vi "Producer Console Entry.vi"(0 "Prod-Data In":T2={"Queue_Producer"=refnum, "Queue_Consumer"=refnum, "To_GUI-Error_message"=refnum, "Rx-Data"=[], "Tx-Data"=[], "Console log"="", "Communication Settings"={"Tx Protocol"=enum."Not Active", "Rx Protocol"=enum."Serial", "Serial"={"Tx Port"="", "Rx Port"="", "Baud rate"=8, "Parity"=enum."Space", "Data bits"=0, "Stop bits"=0, "Flow control"=enum."None", "Tx Resource"="", "Rx Resource"=""}, "MIDI Device"={"Input uDevice ID"=0, "Output uDevice ID"=0, "hmidiout Handle"=0, "hmidiin Handle"=0}, "Bluetooth"={"Dummy"=""}, "USB"={"Dummy"=""}}, "MIDI-Messages"=[], "Queue_Session"=refnum, "To_GUI-Pre-Session"=refnum, "To_GUI-Producer"=refnum, "Tx Info"={"Datatype"=[], "Bytesize"=[], "Strings"=[], "ByteSum"=0}, "Payload"=variant, "Timout-Time[ms]"=0, "To_GUI-Session"=refnum, "CPU(ms)"=0}, 11 "Console Entry":string, 13 "Error In":errorcluster) -> (4 "Prod-Data Out":T2={"Queue_Producer"=refnum, "Queue_Consumer"=refnum, "To_GUI-Error_message"=refnum, "Rx-Data"=[], "Tx-Data"=[], "Console log"="", "Communication Settings"={"Tx Protocol"=enum."Not Active", "Rx Protocol"=enum."Serial", "Serial"={"Tx Port"="", "Rx Port"="", "Baud rate"=8, "Parity"=enum."Space", "Data bits"=0, "Stop bits"=0, "Flow control"=enum."None", "Tx Resource"="", "Rx Resource"=""}, "MIDI Device"={"Input uDevice ID"=0, "Output uDevice ID"=0, "hmidiout Handle"=0, "hmidiin Handle"=0}, "Bluetooth"={"Dummy"=""}, "USB"={"Dummy"=""}}, "MIDI-Messages"=[], "Queue_Session"=refnum, "To_GUI-Pre-Session"=refnum, "To_GUI-Producer"=refnum, "Tx Info"={"Datatype"=[], "Bytesize"=[], "Strings"=[], "ByteSum"=0}, "Payload"=variant, "Timout-Time[ms]"=0, "To_GUI-Session"=refnum, "CPU(ms)"=0})   [LabVIEW 2019]
doc: "Adds a new entry to a console log, if an error has occured it will also be logged."
uses:
  Controls/Producer-Data.ctl
  Common/Controls/Application_Message.ctl
  Common/Controls/Application_State.ctl
  Common/Controls/Communication_Settings.ctl
  Common/Controls/Communication_Protocols.ctl
  MIDI/Controls/MIDI-Message_Array.ctl
  MIDI/Controls/MIDI-Message_Cluster.ctl
  MIDI/Controls/Meta_Commands.ctl
  Controls/Prod - Tx_Info.ctl
panel:
  in  "Tab Control":T1(tab)
  out "Console log in":string
  out "Timestamp":string
  out "Console log out":string
  out "VI-filename":string
  out "VI Path":path
  out "Code Size":u32
  out "Revision Number":u32
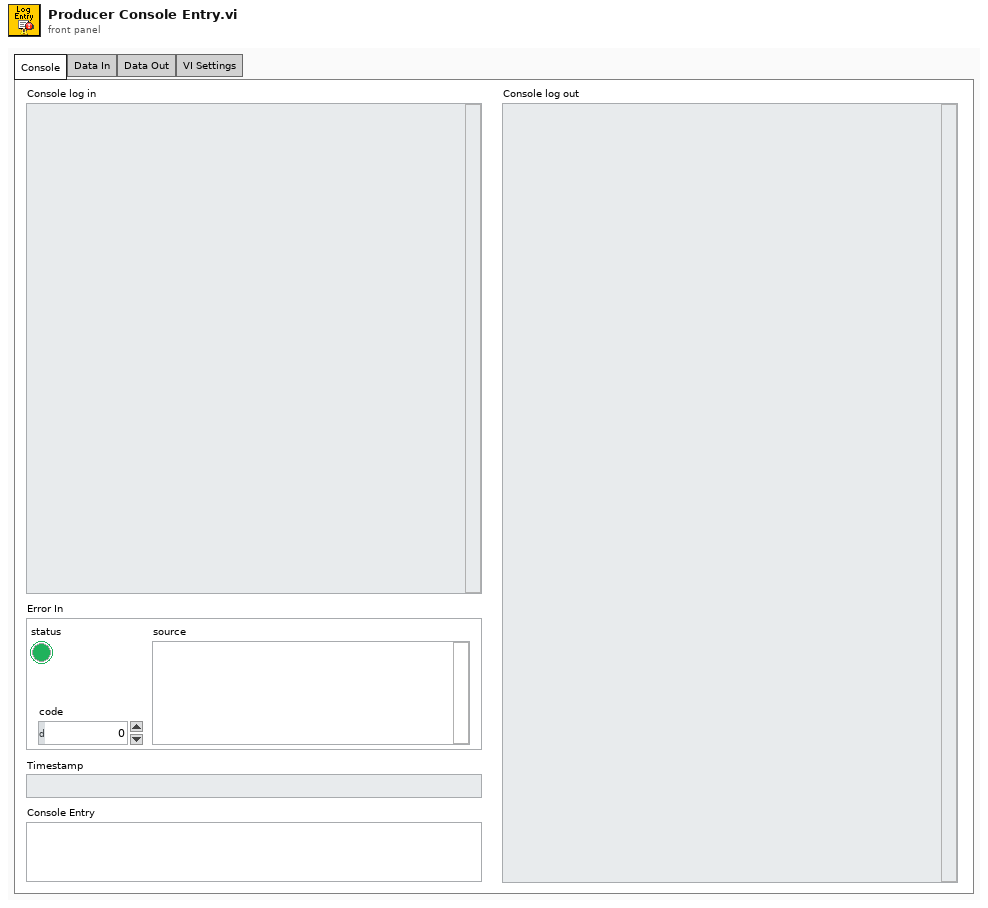
[diagram p1: front panel]
types:
  T1 = enum32{"Console", "Data In", "Data Out", "VI Settings"}
  T2 = typedef "Producer-Data.ctl" = cluster{"Queue_Producer":refnum<queue>, "Queue_Consumer":refnum<queue>, "To_GUI-Error_message":refnum<user-event>, "Rx-Data":i8[], "Tx-Data":i8[], "Console log":string, "Communication Settings":T3, "MIDI-Messages":T5, "Queue_Session":refnum<queue>, "To_GUI-Pre-Session":refnum<user-event>, "To_GUI-Producer":refnum<user-event>, "Tx Info":T8, "Payload":variant, "Timout-Time[ms]":i32, "To_GUI-Session":refnum<user-event>, "CPU(ms)":u32}
  T3 = typedef "Communication_Settings.ctl" = cluster{"Tx Protocol":T4, "Rx Protocol":T4, "Serial":cluster{"Tx Port":refnum<visa-resource-name>, "Rx Port":refnum<visa-resource-name>, "Baud rate":i32, "Parity":enum16{"None", "Odd", "Even", "Mark", "Space"}, "Data bits":i32, "Stop bits":i32, "Flow control":enum16{"None", "XON/XOFF", "RTS/CTS", "XON/XOFF & RTS/CTS", "DTR/DSR", "XON/XOFF & DTR/DSR"}, "Tx Resource":refnum<visa-resource-name>, "Rx Resource":refnum<visa-resource-name>}, "MIDI Device":cluster{"Input uDevice ID":u32, "Output uDevice ID":u32, "hmidiout Handle":i32, "hmidiin Handle":i32}, "Bluetooth":cluster{"Dummy":string}, "USB":cluster{"Dummy":string}}
  T4 = typedef "Communication_Protocols.ctl" = enum16{"Serial", "Bluetooth", "USB-MIDI", "MIDI (Audio Device)", "Not Active"}
  T5 = typedef "MIDI-Message_Array.ctl" = T6[]
  T6 = typedef "MIDI-Message_Cluster.ctl" = cluster{"Message Name":string, "Meta value":i32, "Datastring":string, "Datatype":T7}
  T7 = typedef "Meta_Commands.ctl" = enum16{"No Data", "Pause", "Loop", "Wait for Rx", "Delay", "Break", "MIDI"}
  T8 = typedef "Prod - Tx_Info.ctl" = cluster{"Datatype":T7[], "Bytesize":i32[], "Strings":string[], "ByteSum":i32}
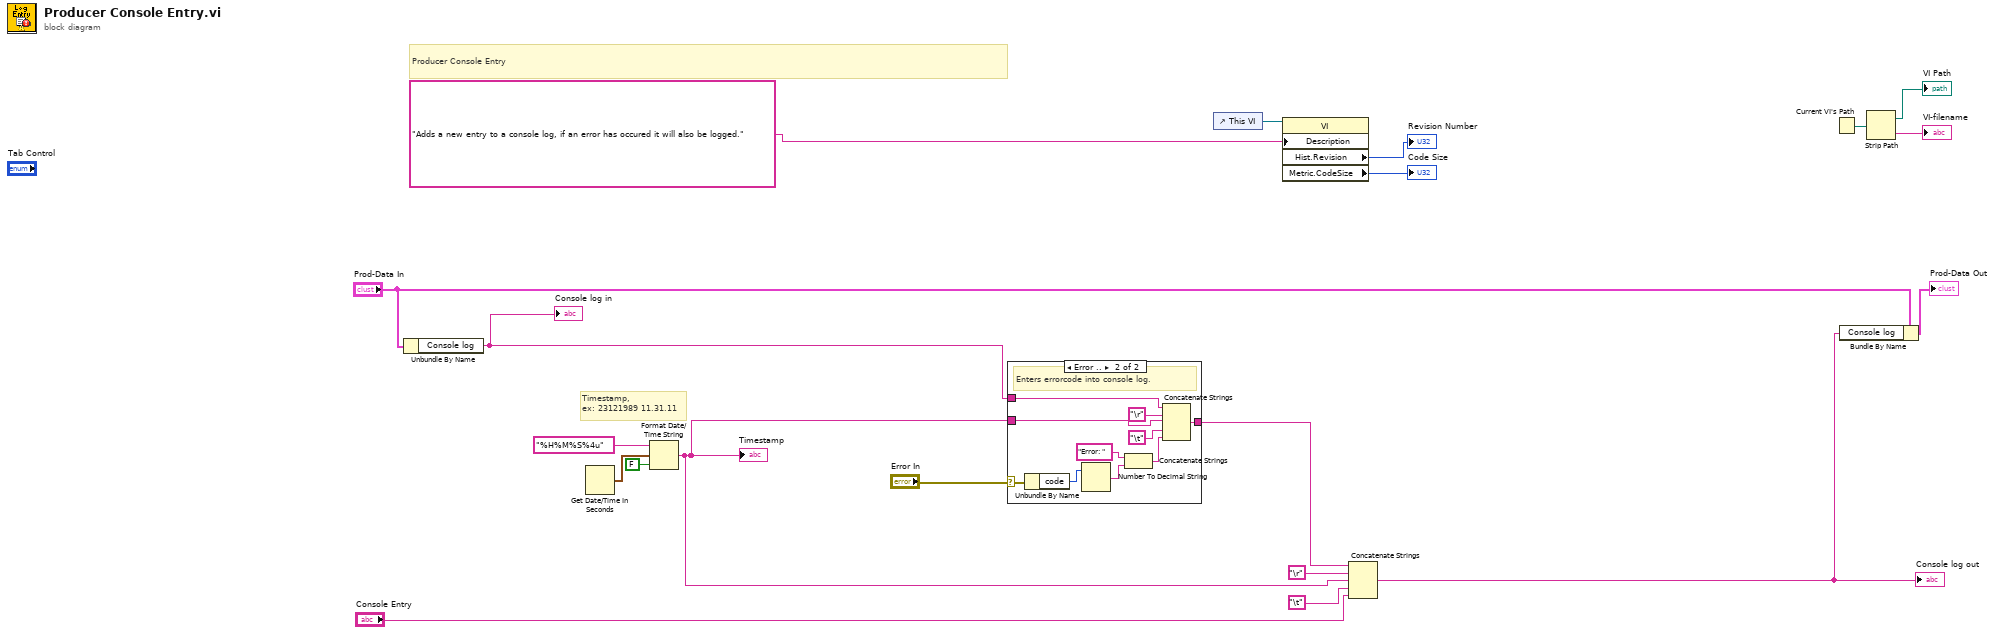
[diagram p0: block diagram]
diagram:
  # "Timestamp, \nex: 23121989 11.31.11"
  # "Producer Console Entry"
  n1 = Unbundle By Name("Prod-Data In") -> ("Console log"=w9:string)
  "Console log in" <- w9
  n2 = Get Date/Time In Seconds() -> (seconds since 1Jan1904=w13:timestamp)
  n3 = Format Date/Time String(time format string (%c)="%H%M%S%4u", seconds (now)=w13, UTC format=FALSE) -> (date/time string=w8:string)
  "Timestamp" <- w8
  n4 = case shown="Error .." "Error In" {
    selector: "Error In" -> [_ w22]
    tunnel: w9 -> [w21 w27]
    tunnel: w8 -> [_ w25]
    tunnel: [w21 w23] -> w7
    frame No Error {
    }
    frame Error {
      # "Enters errorcode into console log."
      n5 = Unbundle By Name(w22) -> ("code"=w31:i32)
      n6 = Number To Decimal String(number=w31) -> (decimal integer string=w30:string)  [unwired: 1 in]
      n7 = Concatenate Strings("Error: " ("string"), w30) -> (w29:string)
      n8 = Concatenate Strings(w27, "\r", w25, "\t", w29) -> (w23:string)
    }
  }
  n9 = control-ref of="This VI"() -> (w4:refnum<vi>)
  n10 = property class="VI"(reference=w4, "Description"="Adds a new entry to a console log, if an error has occured it will also be logged.") -> ("Hist.Revision"=→"Revision Number":u32, "Metric.CodeSize"=→"Code Size":u32)  [unwired: 1 in, 2 out]
  n11 = Concatenate Strings(w7, "\r", w8, "\t", "Console Entry") -> (w16:string)
  "Console log out" <- w16
  n12 = Current VI's Path() -> (path=w20:path)
  n13 = Bundle By Name(cluster="Prod-Data In", "Console log"=w16) -> (→"Prod-Data Out":T2)
  n14 = Strip Path(path=w20) -> (stripped path=→"VI Path":path, name=→"VI-filename":string)
